vi "EvenOdd.vi"() -> ()   [LabVIEW 2022 SP3]
panel:
  in  "?":bool
  out "Iteration":dbl
  out "Even":bool
  out "Odd":bool
  # "EvenOdd:"
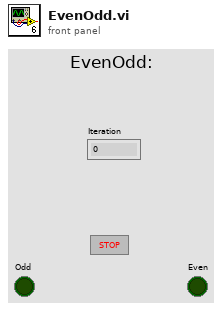
[diagram p1: front panel]
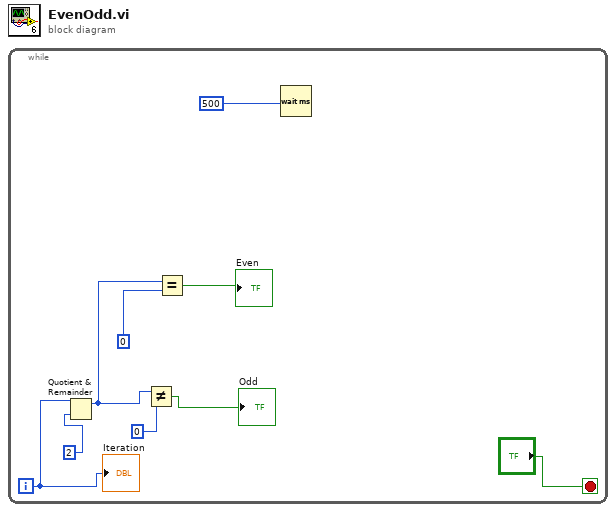
[diagram p0: block diagram]
diagram:
  n1 = while {
    i -> [w2]
    stop <- "?" stop-if-true
    n2 = Quotient & Remainder(x=w2, y=2) -> (x-y*floor(x/y)=w4:i32)  [unwired: 1 out]
    n3 = Not Equal?(x=w4, y=0) -> (x != y?=→"Odd":bool)
    n4 = Equal?(x=w4, y=0) -> (x = y?=→"Even":bool)
    n5 = Wait (ms)(milliseconds to wait=500) -> ()  [unwired: 1 out]
    "Iteration" <- w2
  }
